vi "Test_WriteItem_ReadItem_CorrectValue.vi"(8 "error in (no error)":errorcluster, 11 "TestCase in":refnum<class "TestComposedLookupTable.lvclass">) -> (0 "error out":errorcluster, 3 "TestCase out":refnum<class "TestComposedLookupTable.lvclass">)   [LabVIEW 2017, in "TestComposedLookupTable.lvclass"]
uses:
  TestComposedLookupTable.lvclass
  Source/LookupTable/LookupTable.lvclass/LookupTable.ctl
  3664b224-a50b-4129-af9d-1b8eb270b2f4.vi
  ddd58f5c-5c68-4874-a611-c4c6641c4088.vi
  Source/LookupTable/Read Table Reference.vi
  3664b224-a50b-4129-af9d-1b8eb270b2f4.vi/cf998f27-ad52-476d-abb3-9d149b43456c.vi
  ddd58f5c-5c68-4874-a611-c4c6641c4088.vi/65095b18-87f7-4358-8935-10fd1807acf9.vi
  Source/LookupTable/LookupTable.lvclass
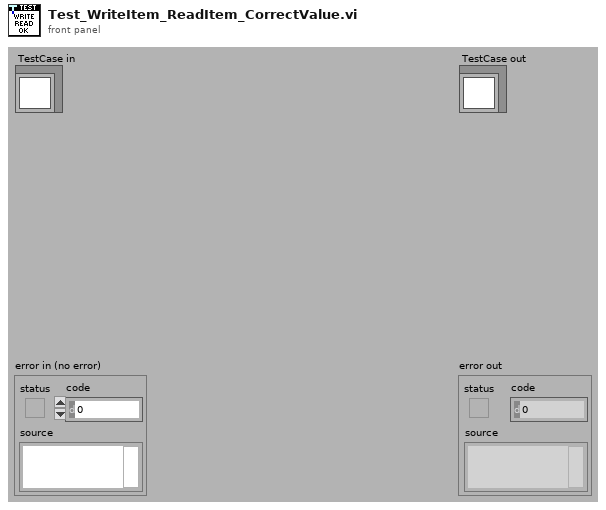
[diagram p1: front panel]
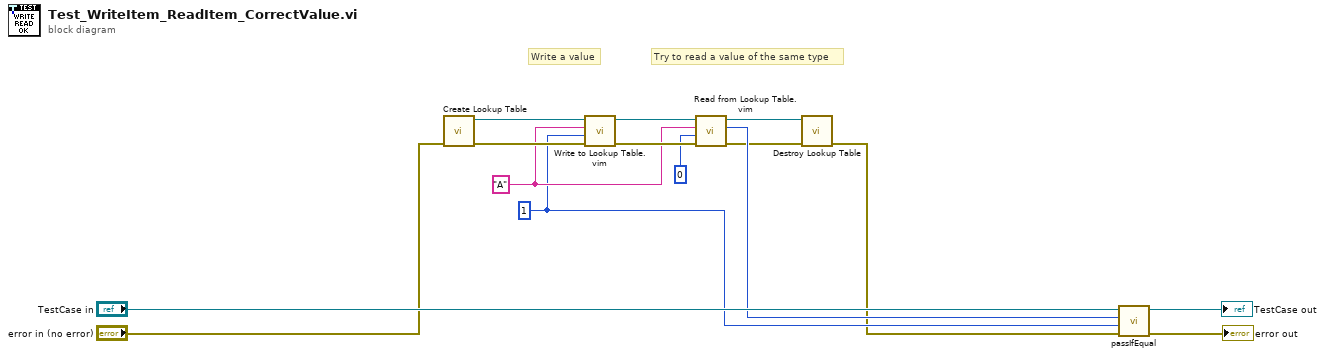
[diagram p0: block diagram]
diagram:
  w7 = 1
  w8 = "A" ("Item Name")
  # "Try to read a value of the same type"
  # "Write a value"
  n1 = call "Create Lookup Table.vi"("error in (no error)"="error in (no error)") -> ("error out"=w15:errorcluster, "LookupTable Reference"=w6:refnum<data-value>)  [unwired: 9 in]
  n2 = call "Write to Lookup Table.vim"("error in (no error)"=w15, "Item"=w7, "Item Name"=w8, "LookupTable Reference"=w6) -> ("error out"=w14:errorcluster, "LookupTable Reference Out"=w9:refnum<data-value>)  [unwired: 5 in, 1 out]
  n3 = call "Read from Lookup Table.vim"("error in (no error)"=w14, "Type"=0, "Item Name"=w8, "LookupTable Reference"=w9) -> ("error out"=w3:errorcluster, "Value"=w10:i32, "LookupTable Reference Out"=w4:refnum<data-value>)  [unwired: 4 in, 1 out]
  n4 = call "Destroy Lookup Table.vi"("error in (no error)"=w3, "LookupTable Reference"=w4) -> ("error out"=w2:errorcluster)  [unwired: 9 in]
  n5 = call-dynamic "passIfEqual.vi"("error in (no error)"=w2, "y"=w7, "x"=w10, "TestCase in"="TestCase in") -> ("error out"=→"error out":errorcluster, "TestCase out"=→"TestCase out":refnum<class "TestComposedLookupTable.lvclass">)  [unwired: 6 in]
